vi "Get Type.vi"(8 "error in (no error)":errorcluster, 11 "Binary Instr in":refnum<class "Binary Instr.lvclass">) -> (0 "error out":errorcluster, 2 "Type":string, 3 "Binary Instr out":refnum<class "Binary Instr.lvclass">)   [LabVIEW 2015, in "Item Actor.lvlib" / "Binary Instr.lvclass"]
uses:
  Binary Instr.lvclass
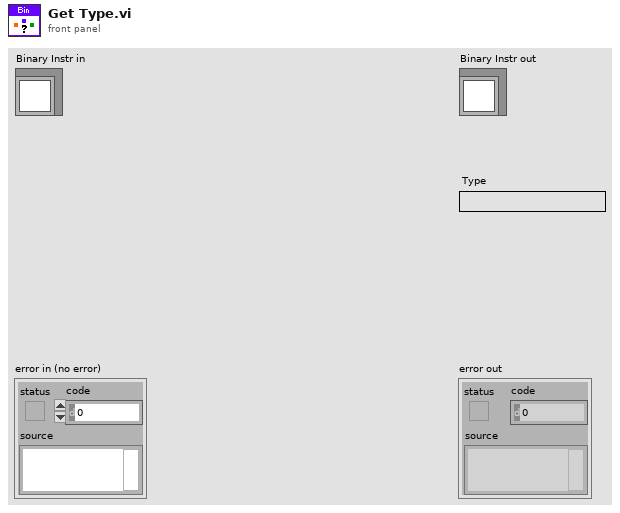
[diagram p1: front panel]
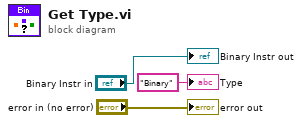
[diagram p0: block diagram]
diagram:
  "error out" <- "error in (no error)"
  "Binary Instr out" <- "Binary Instr in"
  "Type" <- "Binary" ("Type")
